vi "getAll.vi"(8 "error in (no error)":errorcluster, 11 "instrument.PPMS1 in":refnum<class "instrument.PPMS1.lvclass">) -> (0 "error out":errorcluster, 2 "getAll":variant, 3 "instrument.PPMS1 out":refnum<class "instrument.PPMS1.lvclass">)   [LabVIEW 2019, in "instrument.PPMS1.lvclass"]
uses:
  instrument.PPMS1.lvclass
  C:/Users/patrick/Documents/GitHub/PPMS-Monitor-and-Control/lvsrc/instrument.PPMS/instrument.PPMS.lvclass
  instrument.PPMS/Typedefs/PPMS.getAll--cluster.ctl
  instrument.PPMS/instrument.PPMS.lvclass
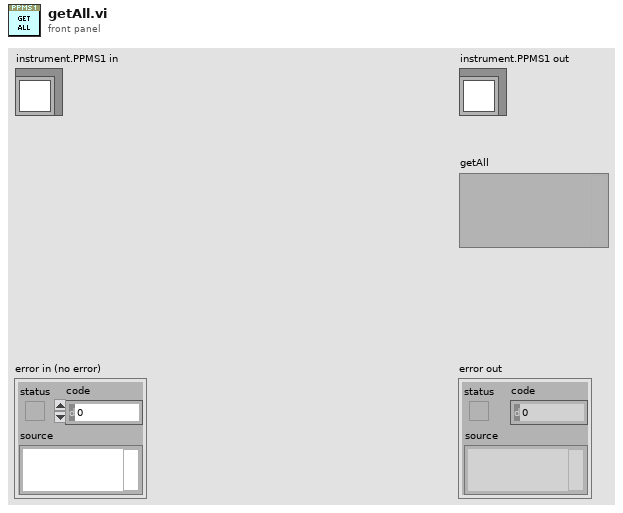
[diagram p1: front panel]
types:
  T1 = typedef "instrument.PPMS.lvclass/PPMS.getAll--cluster.ctl" = cluster{"Helium Level (%)":dbl, "Temperature (K)":dbl, "Temperature Status":string, "Magnetic Field (T)":dbl, "Magnet Status":string, "Position (°)":dbl}
  T2 = typedef "instrument.PPMS.lvclass/PPMS.Temperature Status--cluster.ctl" = cluster{"Temperature (K)":dbl, "Temperature Status":string}
  T3 = typedef "instrument.PPMS.lvclass/PPMS.Magnet Status--cluster.ctl" = cluster{"Field (T)":dbl, "Magnet Status":string}
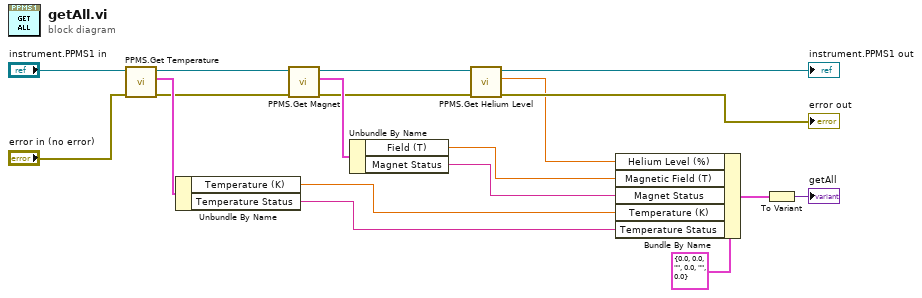
[diagram p0: block diagram]
diagram:
  n1 = call "PPMS.Get Temperature.vi"("error in (no error)"="error in (no error)", "instrument.PPMS"="instrument.PPMS1 in") -> ("error out"=w12:errorcluster, "Temperature Status"=w14:T2, "instrument.PPMS out"=w16:refnum<class "instrument.PPMS1.lvclass">)  [unwired: 7 in]
  n2 = Unbundle By Name(w14) -> ("Temperature (K)"=w6:dbl, "Temperature Status"=w5:string)
  n3 = call "PPMS.Get Magnet.vi"("error in (no error)"=w12, "instrument.PPMS"=w16) -> ("error out"=w11:errorcluster, "Magnet Status"=w13:T3, "instrument.PPMS out"=w15:refnum<class "instrument.PPMS1.lvclass">)  [unwired: 7 in]
  n4 = Unbundle By Name(w13) -> ("Field (T)"=w3:dbl, "Magnet Status"=w4:string)
  n5 = call "PPMS.Get Helium Level.vi"("error in (no error)"=w11, "instrument.PPMS"=w15) -> ("error out"=→"error out":errorcluster, "Helium Level (%)"=w2:dbl, "instrument.PPMS out"=→"instrument.PPMS1 out":refnum<class "instrument.PPMS1.lvclass">)  [unwired: 7 in]
  n6 = Bundle By Name(cluster=T1 {"Helium Level (%)"=0.0, "Temperature (K)"=0.0, "Temperature Status"="", "Magnetic Field (T)"=0.0, "Magnet Status"="", "Position (°)"=0.0} ("getAll"), "Helium Level (%)"=w2, "Magnetic Field (T)"=w3, "Magnet Status"=w4, "Temperature (K)"=w6, "Temperature Status"=w5) -> (w17:T1)
  n7 = To Variant(anything=w17) -> (Variant=→"getAll":variant)
